vi "Configure test.vi"(6 "Assert VI Path":path, 7 "Existing Queue Elements":string, 8 "error in (no error)":errorcluster, 11 "Basic Int LT in":refnum<class "Int LT.lvclass">) -> (0 "error out":errorcluster, 3 "Basic Int LT out":refnum<class "Int LT.lvclass">)   [LabVIEW 2018, in "Int LT.lvclass"]
uses:
  Int LT.lvclass
  fe0e7bb0-81a2-4c30-80a4-bef1744cb67d.vi
  <vilib>/JDP Science/JSONtext/Find Item.vi
  fe0e7bb0-81a2-4c30-80a4-bef1744cb67d.vi/6c529ba6-ed1d-4692-bf5f-6d1820cf2dc4.vi
  fe0e7bb0-81a2-4c30-80a4-bef1744cb67d.vi/4a40591f-342d-490c-b9c7-482cc62b07ba.vi
  <vilib>/JDP Science/JSONtext/String Subset.vi
  Test Class String IDs.vi
  <vilib>/JDP Science/JSONtext/Parsing/Parse Full Path or Item Name.vi
  <vilib>/JDP Science/JSONtext/Offset/Find Item Locations by Path.vi
  <vilib>/JDP Science/JSONtext/JSON text to Variant.vi
  <vilib>/JDP Science/JSONtext/Variant to JSON Text.vi
  <vilib>/JDP Science/JSONtext/Set Item.vi
  Integer.lvclass
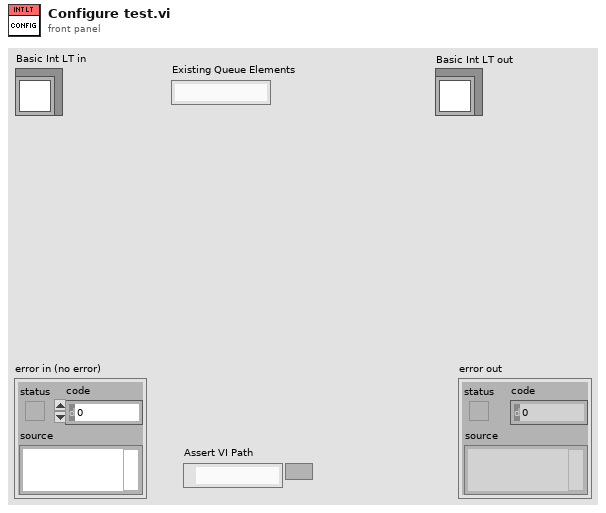
[diagram p1: front panel]
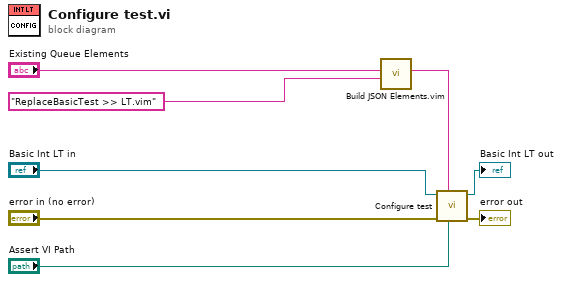
[diagram p0: block diagram]
diagram:
  n1 = call "Build JSON Elements.vim"("Append Element(s)"="ReplaceBasicTest >> LT.vim", "JSON Elements in ({})"="Existing Queue Elements") -> ("JSON Elements out"=w1:string)  [unwired: 9 in]
  n2 = call-parent "Configure test.vi"("Assert VI Path"="Assert VI Path", "Existing Queue Elements"=w1, "error in (no error)"="error in (no error)", "Basic Integer in"="Basic Int LT in") -> ("error out"=→"error out":errorcluster, "Basic Integer out"=→"Basic Int LT out":refnum<class "Int LT.lvclass">)  [unwired: 6 in]
